vi "Read Events.vi"(11 "Cooler UI with Events in":refnum<class "Cooler UI with Events.lvclass">) -> (2 "Events":T1, 3 "Cooler UI with Events out":refnum<class "Cooler UI with Events.lvclass">)   [LabVIEW 2012, in "Cooler UI.lvlib" / "Cooler UI with Events.lvclass"]
uses:
  Cooler UI with Events.lvclass
  Events.ctl
  Cooler UI with Events.lvclass/Cooler UI with Events.ctl
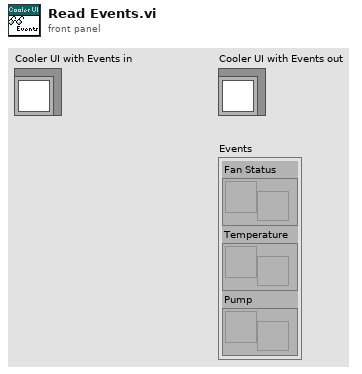
[diagram p1: front panel]
types:
  T1 = typedef "Cooler UI.lvlib/Cooler UI with Events.lvclass/Events.ctl" = cluster{"Fan Status":refnum<user-event>, "Temperature":refnum<user-event>, "Pump":refnum<user-event>}
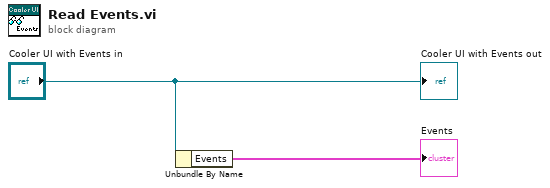
[diagram p0: block diagram]
diagram:
  n1 = Unbundle By Name("Cooler UI with Events in") -> ("Events"=→"Events":T1)
  "Cooler UI with Events out" <- "Cooler UI with Events in"
